vi "SLM_CalibratorOnly1.vi"() -> ()   [LabVIEW 2011]
uses:
  <vilib>/userDefined/High Color/IMAQdx.ctl
  <vilib>/vision/driver/NI_Vision_Acquisition_Software.lvlib
  <vilib>/vision/NI_Vision_Development_Module.lvlib
panel:
  in  "Step:":i32=4
  in  "Boolean":bool caption="SLM1"
  in  "path":path=path "C:/Users/Lab541/Documents/BAUL - TRASH/070214_SLM2" caption="Folder to save data"
  in  "STOP":bool
  out "CCD":T1(plugin-control)
  out "SupportFiles path":path
  in  "Ready?\nCalibrate!":bool caption="Stop (F)"
  in  "Active2":bool=TRUE caption="Hide/Show (Show)"
  in  "Active1":bool=TRUE caption="Hide/Show (Show)"
  in  "Yc1":dbl(slide)=1.3147410358565736 scale=0.0..10.0
  in  "Yf1:":dbl(slide)=2.8685258964143427 caption="Fine:" scale=0.0..10.0
  in  "Xc1":dbl(slide)=9.664429530201343 caption="X position" scale=0.0..10.0
  in  "Xf1:":dbl(slide)=9.664429530201343 caption="Fine:" scale=0.0..10.0
  out "Yi1":dbl caption="Y position"
  out "Xi1":dbl
  in  "Xc2":dbl(slide)=1.4429530201342282 caption="X position" scale=0.0..10.0
  in  "Xf2:":dbl(slide)=6.10738255033557 caption="Fine:" scale=0.0..10.0
  out "Xi2":dbl
  in  "Yf2:":dbl(slide)=5.467625899280575 caption="Fine:" scale=0.0..10.0
  in  "Yc2":dbl(slide)=3.598326359832636 scale=0.0..10.0
  out "Yi2":dbl caption="Y position"
  out "CGH_x\nSLM1":T1(plugin-control)
  out "CGH_y\nSLM2":T1(plugin-control)
  in  "Gradient1":bool
  in  "Gradient2":bool
  out "Status:":string
  in  "Label:":string
  out "Images done":dbl(slide) scale=0.0..256.0
  # "SLM2"
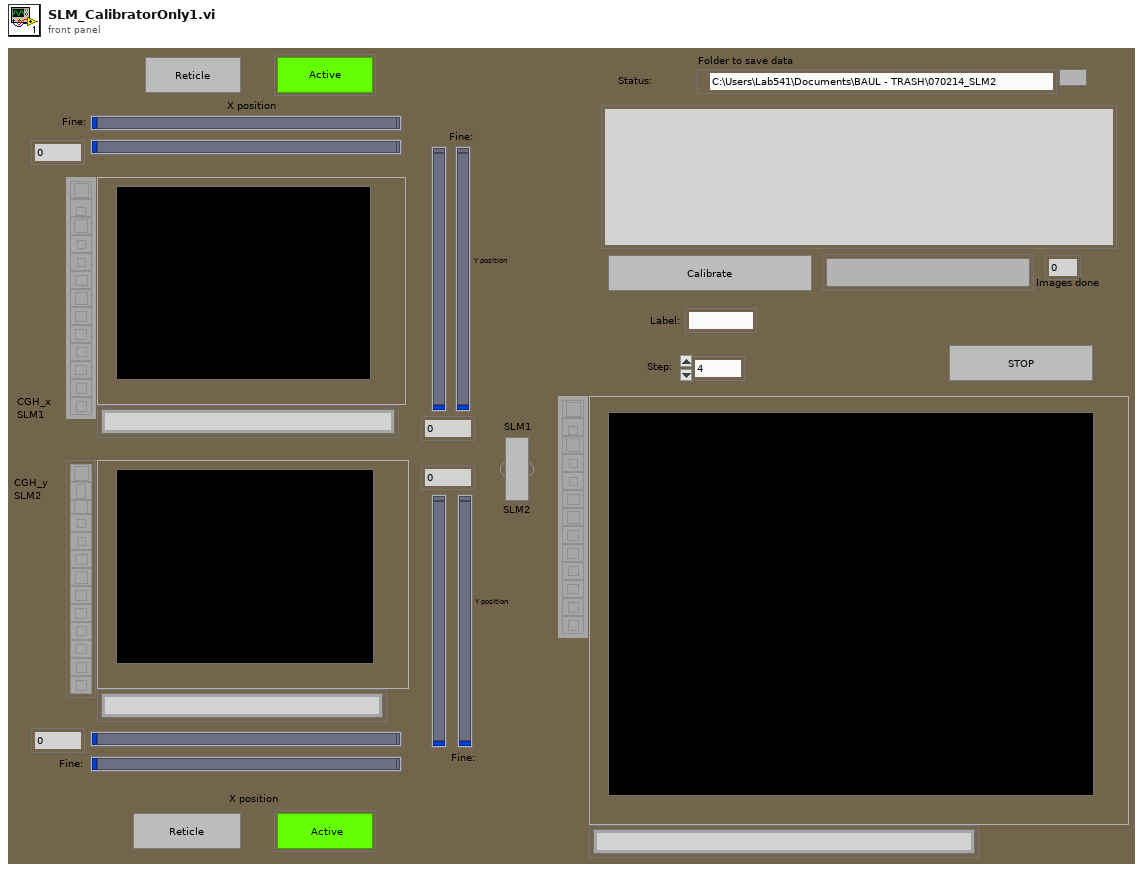
[diagram p1: front panel]
types:
  T1 = typedef "IMAQ Image.ctl" = refnum<image>
  T2 = typedef "IMAQdx.ctl" = refnum<k21>
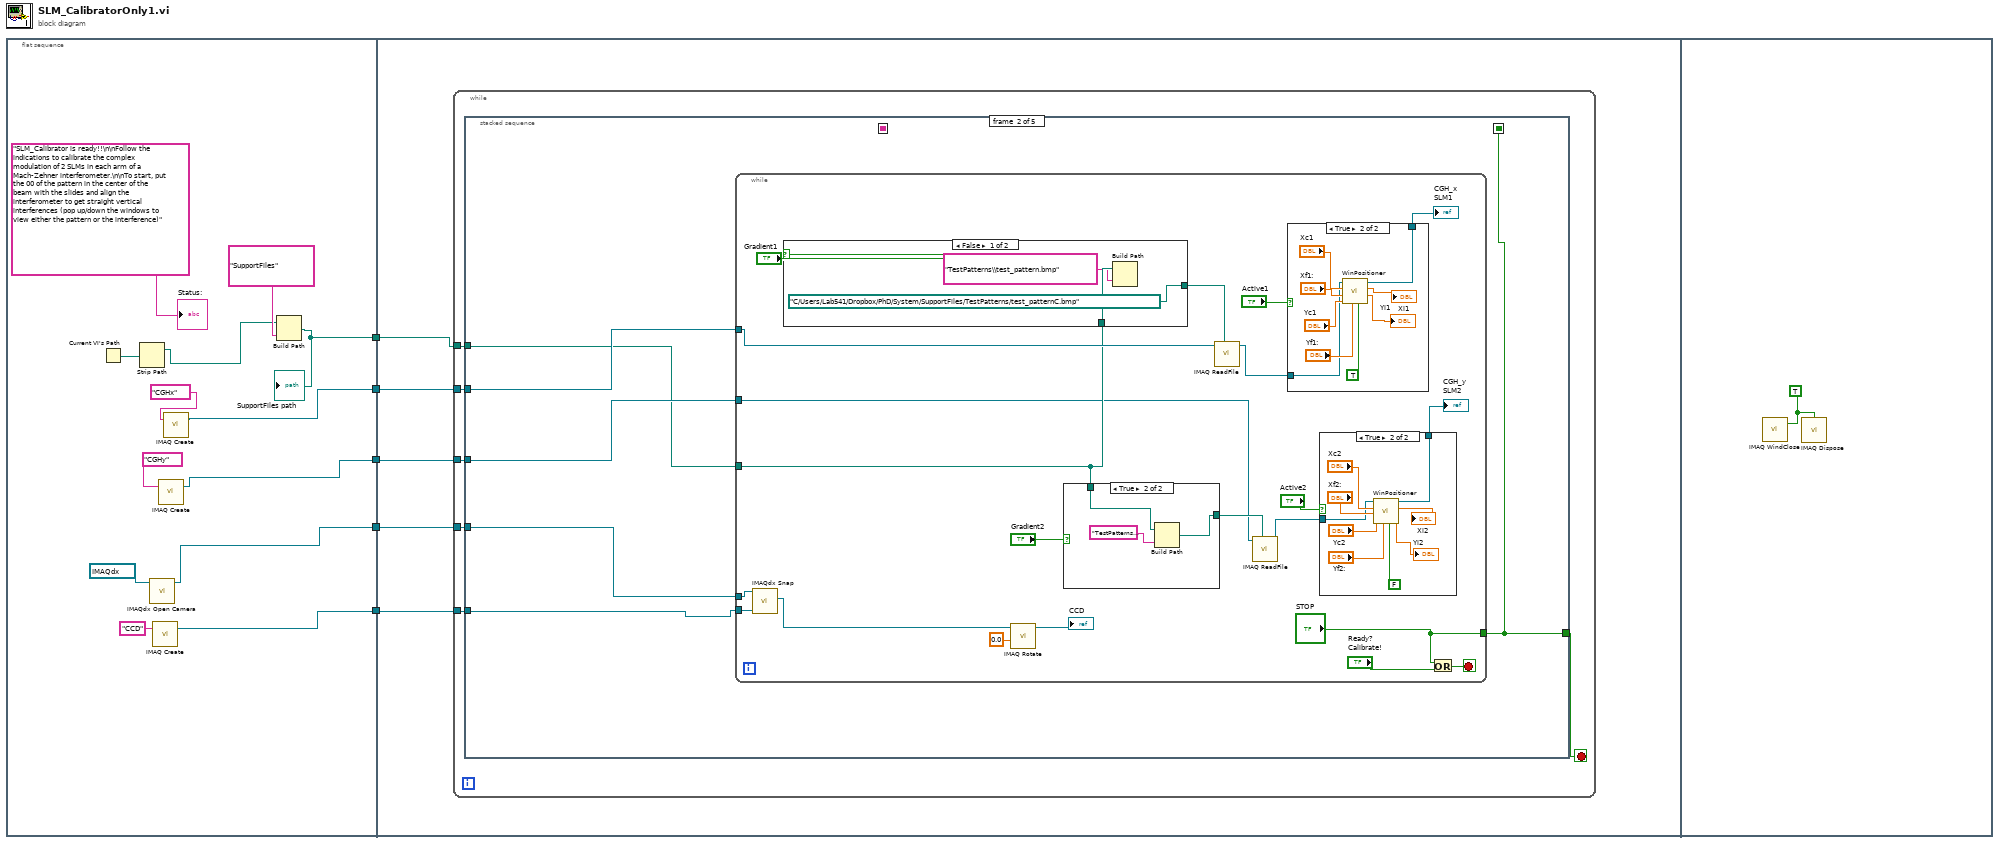
[diagram p0: block diagram]
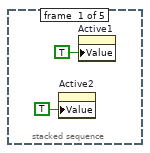
[diagram p2: hidden frame]
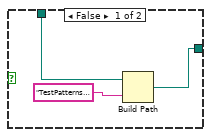
[diagram p3: hidden frame]
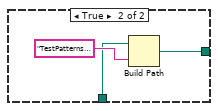
[diagram p4: hidden frame]
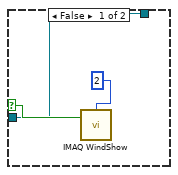
[diagram p5: hidden frame]
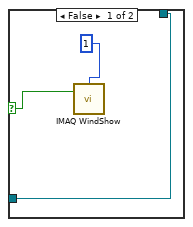
[diagram p6: hidden frame]
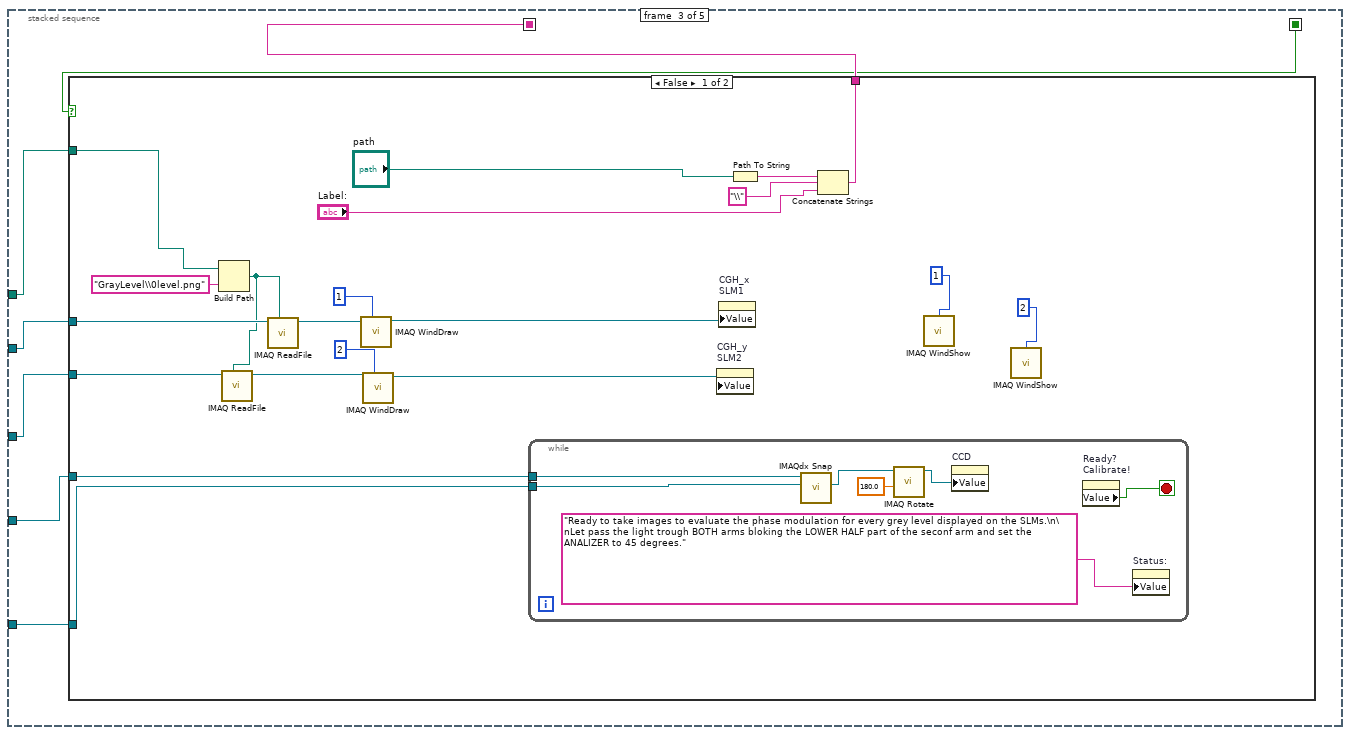
[diagram p7: hidden frame]
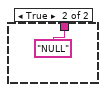
[diagram p8: hidden frame]
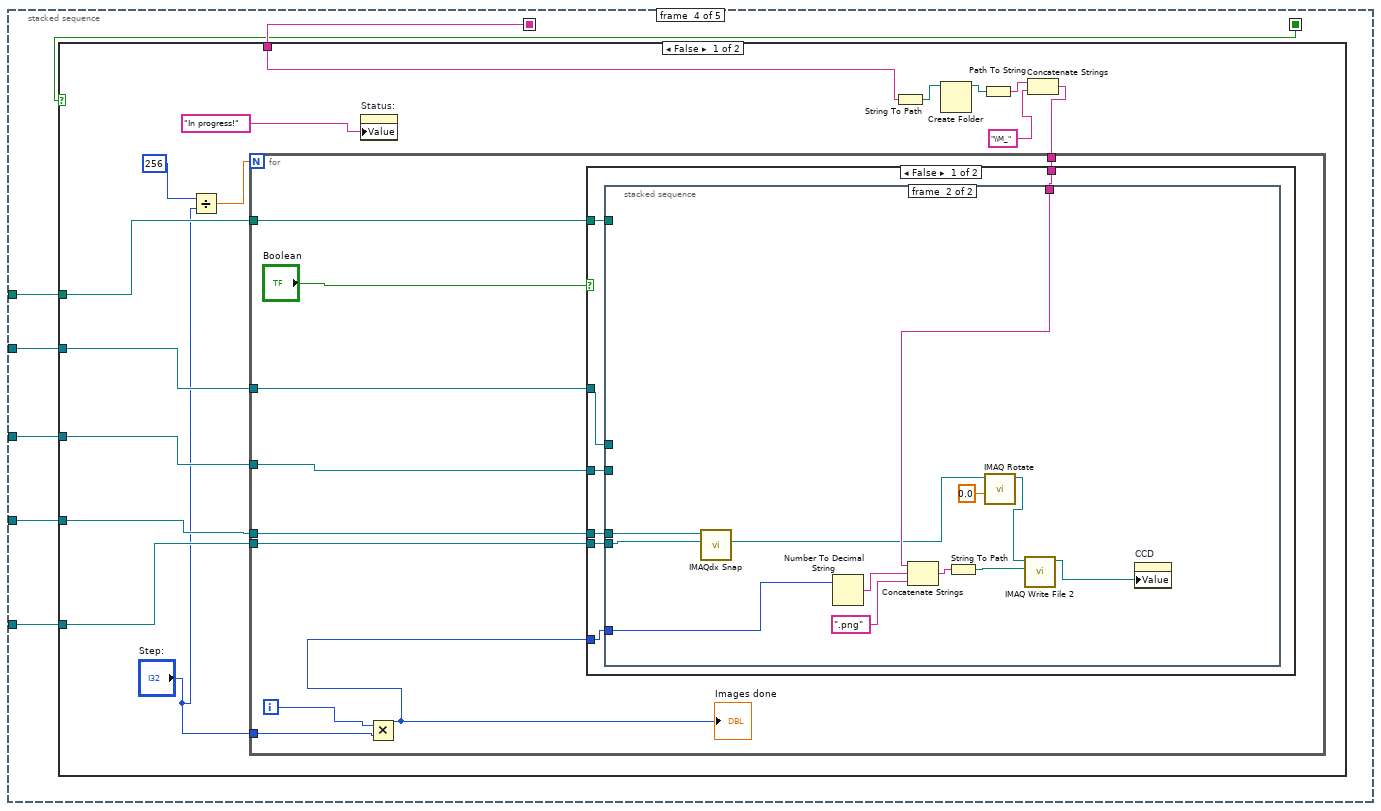
[diagram p9: hidden frame]
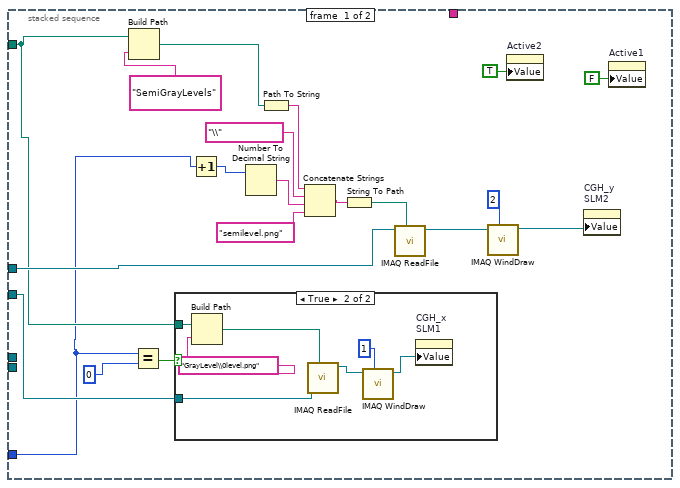
[diagram p10: hidden frame]
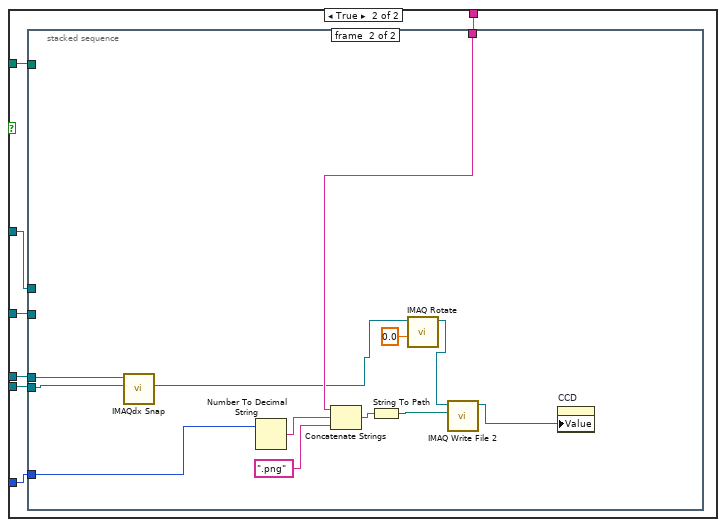
[diagram p12: hidden frame]
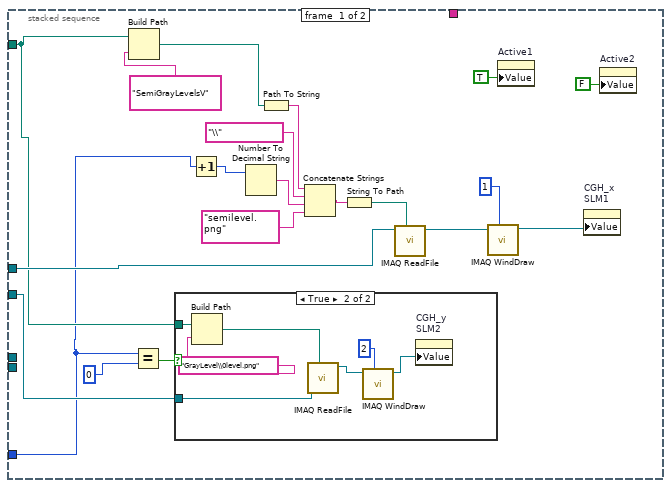
[diagram p13: hidden frame]
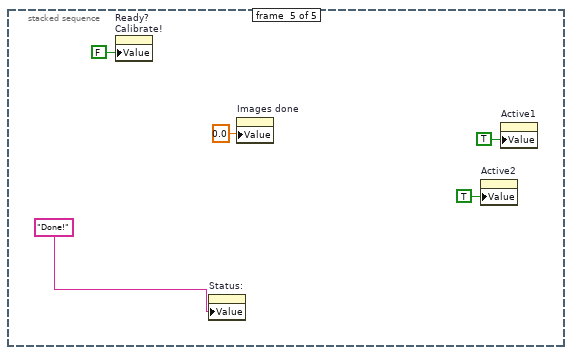
[diagram p16: hidden frame]
diagram:
  n1 = flat-sequence {
    tunnel: [w10] -> w5
    tunnel: [w9] -> w4
    tunnel: [w8] -> w3
    tunnel: [w7] -> w2
    tunnel: [w6] -> w1
    tunnel: w5 -> [w23]
    tunnel: w4 -> [w22]
    tunnel: w3 -> [w21]
    tunnel: w2 -> [w20]
    tunnel: w1 -> [w19]
    frame #0 {
      n2 = Current VI's Path() -> (path=w14:path)
      n3 = Strip Path(path=w14) -> (stripped path=w15:path)  [unwired: 1 out]
      n4 = call <vilib>:"IMAQdx Open Camera.vi"("Session In"=T2 "cam0") -> ("Session Out"=w7:T2)  [unwired: 9 in, 1 out]
      n5 = call "IMAQ Create"("Image Name"="CCD") -> ("New Image"=w6:T1)  [unwired: 4 in, 1 out]
      n6 = call "IMAQ Create"("Image Name"="CGHy") -> ("New Image"=w8:T1)  [unwired: 4 in, 1 out]
      n7 = call "IMAQ Create"("Image Name"="CGHx") -> ("New Image"=w9:T1)  [unwired: 4 in, 1 out]
      n8 = Build Path(base path=w15, name or relative path="SupportFiles") -> (appended path=w10:path)
      "SupportFiles path" <- w10
      "Status:" <- "SLM_Calibrator is ready!!\n\nFollow the indications to calibrate the complex modulation of 2 SLMs in each arm of a Mach-Zehner interferometer.\n\nTo start, put the 00 of the pattern in the center of the beam with the slides and align the interferometer to get straight vertical interferences (pop up/down the windows to view either the pattern or the interference)" ("String")
    }
    frame #1 {
      n9 = while {
        tunnel: w22 -> [w29]
        tunnel: w21 -> [w28]
        tunnel: w19 -> [w27]
        tunnel: w20 -> [w26]
        tunnel: w23 -> [w25]
        stop <- w24 stop-if-true
        n10 = stacked-sequence {
          seq-local: [_ _ w101 _ _] -> [_ _ _ w134 _]
          seq-local: [_ w32 _ _ _] -> [_ _ w95 w130 _]
          tunnel: w28 -> [_ w36 w97 w135 _]
          tunnel: w29 -> [_ w37 w98 w136 _]
          tunnel: w25 -> [_ w35 w99 w133 _]
          tunnel: w27 -> [_ w34 w100 w131 _]
          tunnel: w26 -> [_ w33 w96 w132 _]
          tunnel: [_ w32 _ _ _] -> w24
          frame #0 {
            n11 = property on="Active2" class="Bool (strict)"("Value"=TRUE ("Active1")) -> ()  [unwired: 2 in, 2 out]
            n12 = property on="Active1" class="Bool (strict)"("Value"=TRUE ("Active1")) -> ()  [unwired: 2 in, 2 out]
          }
          frame #1 {
            n13 = while {
              tunnel: w33 -> [w58]
              tunnel: w34 -> [w57]
              tunnel: w37 -> [w51]
              tunnel: w36 -> [w42]
              tunnel: w35 -> [w46]
              tunnel: ["STOP"] -> w32
              stop <- w55 stop-if-true
              n14 = call <vilib>:"IMAQdx Snap.vi"("Image In"=w57, "Session In"=w58) -> ("Image Out"=w40:T1)  [unwired: 7 in, 2 out]
              n15 = case shown="False" "Gradient1" {
                tunnel: w46 -> [w67 w69]
                tunnel: [path "C:/Users/Lab541/Dropbox/PhD/System/SupportFiles/TestPatterns/test_patternC.bmp" ("appended path") w68] -> w47
                frame False {
                  n16 = Build Path(base path=w67, name or relative path="TestPatterns\\test_pattern.bmp") -> ()  [unwired: 1 out]
                }
                frame True {
                  n17 = Build Path(base path=w69, name or relative path="TestPatterns\\test_pattern2V.png") -> (appended path=w68:path)
                }
              }
              n18 = call "IMAQ Rotate"("Angle (degrees)"=sgl 0.0, "Image Src"=w40) -> ("Image Dst Out"=→"CCD":T1)  [unwired: 8 in, 1 out]
              n19 = case shown="True" "Gradient2" {
                tunnel: [w60 w62] -> w44
                tunnel: w46 -> [w59 w63]
                frame False {
                  n20 = Build Path(base path=w59, name or relative path="TestPatterns\\test_pattern.bmp") -> (appended path=w60:path)
                }
                frame True {
                  n21 = Build Path(base path=w63, name or relative path="TestPatterns\\test_pattern2.png") -> (appended path=w62:path)
                }
              }
              n22 = call "IMAQ ReadFile"("File Path"=w47, "Image"=w51) -> ("Image Out"=w43:T1)  [unwired: 5 in, 4 out]
              n23 = call "IMAQ ReadFile"("File Path"=w44, "Image"=w42) -> ("Image Out"=w52:T1)  [unwired: 5 in, 4 out]
              n24 = case shown="True" "Active1" {
                selector: "Active1" -> [w85 _]
                tunnel: [w83 w86] -> w50
                tunnel: w43 -> [w83 w87]
                frame False {
                  n25 = call "IMAQ WindShow"("Hide/Show (Show)"=w85, "Window Number (0...15)"=1) -> ()  [unwired: 4 in, 3 out]
                }
                frame True {
                  n26 = call "WinPositioner.vi"("Image"=w87, "X position"="Xc1", "Fine X position"="Xf1:", "Y position"="Yc1", "Fine Y position"="Yf1:", "Display?"=TRUE) -> ("CGH_x"=w86:T1, "X position"=→"Xi1":dbl, "Y position"=→"Yi1":dbl)  [unwired: 2 in]
                }
              }
              "CGH_x\nSLM1" <- w50
              n27 = case shown="True" "Active2" {
                selector: "Active2" -> [w73 _]
                tunnel: [w71 w74] -> w53
                tunnel: w52 -> [w71 w75]
                frame False {
                  n28 = call "IMAQ WindShow"("Hide/Show (Show)"=w73, "Window Number (0...15)"=2) -> ()  [unwired: 4 in, 3 out]
                }
                frame True {
                  n29 = call "WinPositioner.vi"("Image"=w75, "X position"="Xc2", "Fine X position"="Xf2:", "Y position"="Yc2", "Fine Y position"="Yf2:", "Display?"=FALSE) -> ("CGH_x"=w74:T1, "X position"=→"Xi2":dbl, "Y position"=→"Yi2":dbl)  [unwired: 2 in]
                }
              }
              "CGH_y\nSLM2" <- w53
              n30 = Or(x="STOP", y="Ready?\nCalibrate!") -> (x .or. y?=w55:bool)
            }
          }
          frame #2 {
            n31 = case shown="False" w95 {
              tunnel: [w118 "NULL"] -> w101
              tunnel: w100 -> [w117 _]
              tunnel: w99 -> [w112 _]
              tunnel: w98 -> [w107 _]
              tunnel: w97 -> [w104 _]
              tunnel: w96 -> [w103 _]
              frame False {
                n32 = Build Path(base path=w112, name or relative path="GrayLevel\\0level.png") -> (appended path=w105:path)
                n33 = call "IMAQ ReadFile"("File Path"=w105, "Image"=w104) -> ("Image Out"=w106:T1)  [unwired: 5 in, 4 out]
                n34 = call "IMAQ ReadFile"("File Path"=w105, "Image"=w107) -> ("Image Out"=w108:T1)  [unwired: 5 in, 4 out]
                n35 = call "IMAQ WindDraw"("Window Number (0...15)"=1, "Image"=w108) -> ("Image Out (duplicate)"=w113:T1)  [unwired: 8 in, 1 out]
                n36 = call "IMAQ WindDraw"("Window Number (0...15)"=2, "Image"=w106) -> ("Image Out (duplicate)"=w109:T1)  [unwired: 8 in, 1 out]
                n37 = while {
                  tunnel: w103 -> [w127]
                  tunnel: w117 -> [w126]
                  stop <- w125 stop-if-true
                  n38 = call <vilib>:"IMAQdx Snap.vi"("Image In"=w126, "Session In"=w127) -> ("Image Out"=w123:T1)  [unwired: 7 in, 2 out]
                  n39 = call "IMAQ Rotate"("Angle (degrees)"=sgl 180.0, "Image Src"=w123) -> ("Image Dst Out"=w122:T1)  [unwired: 8 in, 1 out]
                  n40 = property on="CCD" class="ImageControl"("Value"=w122) -> ()  [unwired: 2 in, 2 out]
                  n41 = property on="Ready?\nCalibrate!" class="Bool (strict)"() -> ("Value"=w125:bool)  [unwired: 2 in, 2 out]
                  n42 = property on="Status:" class="Str"("Value"="Ready to take images to evaluate the phase modulation for every grey level displayed on the SLMs.\n\nLet pass the light trough BOTH arms bloking the LOWER HALF part of the seconf arm and set the ANALIZER to 45 degrees." ("message")) -> ()  [unwired: 2 in, 2 out]
                }
                n43 = property on="CGH_y\nSLM2" class="ImageControl"("Value"=w109) -> ()  [unwired: 2 in, 2 out]
                n44 = property on="CGH_x\nSLM1" class="ImageControl"("Value"=w113) -> ()  [unwired: 2 in, 2 out]
                n45 = Path To String(path="path") -> (string=w121:string)
                n46 = Concatenate Strings(w121, "\\" ("string"), "Label:") -> (w118:string)
                n47 = call "IMAQ WindShow"("Window Number (0...15)"=1) -> ()  [unwired: 5 in, 3 out]
                n48 = call "IMAQ WindShow"("Window Number (0...15)"=2) -> ()  [unwired: 5 in, 3 out]
              }
              frame True {
              }
            }
          }
          frame #3 {
            n49 = case shown="False" w130 {
              tunnel: w136 -> [w151 _]
              tunnel: w135 -> [w150 _]
              tunnel: w134 -> [w144 _]
              tunnel: w133 -> [w142 _]
              tunnel: w132 -> [w141 _]
              tunnel: w131 -> [w143 _]
              frame False {
                n50 = Divide(x=256, y="Step:") -> (x/y=w138:dbl)
                n51 = property on="Status:" class="Str"("Value"="In progress!" ("Status")) -> ()  [unwired: 2 in, 2 out]
                n52 = String To Path(string=w144) -> (path=w148:path)
                n53 = Create Folder(path (use dialog)=w148) -> (created path=w147:path)  [unwired: 2 in, 2 out]
                n54 = Path To String(path=w147) -> (string=w146:string)
                n55 = Concatenate Strings(w146, "\\M_") -> (w137:string)
                n56 = for {
                  N: w138 -> [_]
                  tunnel: w151 -> [w161]
                  tunnel: w150 -> [w160]
                  tunnel: w137 -> [w159]
                  tunnel: w142 -> [w158]
                  tunnel: w141 -> [w157]
                  tunnel: w143 -> [w156]
                  tunnel: "Step:" -> [w152]
                  i -> [w155]
                  n57 = Multiply(x=w155, y=w152) -> (x*y=w154:i32)
                  "Images done" <- w154
                  n58 = case shown="False" "Boolean" {
                    tunnel: w161 -> [w162 w213]
                    tunnel: w160 -> [w168 w212]
                    tunnel: w159 -> [w167 w209]
                    tunnel: w158 -> [w166 w214]
                    tunnel: w157 -> [w165 w211]
                    tunnel: w156 -> [w164 w210]
                    tunnel: w154 -> [w163 w208]
                    frame False {
                      n59 = stacked-sequence {
                        tunnel: w163 -> [w171 w203]
                        tunnel: w162 -> [w188 _]
                        tunnel: w168 -> [w173 _]
                        tunnel: w167 -> [_ w202]
                        tunnel: w166 -> [w174 _]
                        tunnel: w165 -> [_ w201]
                        tunnel: w164 -> [_ w200]
                        frame #0 {
                          n60 = Build Path(base path=w174, name or relative path="SemiGrayLevels") -> (appended path=w175:path)
                          n61 = Equal?(x=w171, y=0) -> (x = y?=w178:bool)
                          n62 = case shown="True" w178 {
                            tunnel: w173 -> [_ w193]
                            tunnel: w174 -> [_ w192]
                            frame False {
                            }
                            frame True {
                              n63 = Build Path(base path=w192, name or relative path="GrayLevel\\0level.png") -> (appended path=w190:path)
                              n64 = call "IMAQ ReadFile"("File Path"=w190, "Image"=w193) -> ("Image Out"=w195:T1)  [unwired: 5 in, 4 out]
                              n65 = call "IMAQ WindDraw"("Window Number (0...15)"=1, "Image"=w195) -> ("Image Out (duplicate)"=w189:T1)  [unwired: 8 in, 1 out]
                              n66 = property on="CGH_x\nSLM1" class="ImageControl"("Value"=w189) -> ()  [unwired: 2 in, 2 out]
                            }
                          }
                          n67 = Increment(x=w171) -> (x+1=w182:i32)
                          n68 = Number To Decimal String(number=w182) -> (decimal integer string=w183:string)  [unwired: 1 in]
                          n69 = Path To String(path=w175) -> (string=w184:string)
                          n70 = Concatenate Strings(w184, "\\", w183, "semilevel.png") -> (w180:string)
                          n71 = String To Path(string=w180) -> (path=w179:path)
                          n72 = call "IMAQ ReadFile"("File Path"=w179, "Image"=w188) -> ("Image Out"=w187:T1)  [unwired: 5 in, 4 out]
                          n73 = call "IMAQ WindDraw"("Window Number (0...15)"=2, "Image"=w187) -> ("Image Out (duplicate)"=w172:T1)  [unwired: 8 in, 1 out]
                          n74 = property on="Active2" class="Bool (strict)"("Value"=TRUE ("Active1")) -> ()  [unwired: 2 in, 2 out]
                          n75 = property on="CGH_y\nSLM2" class="ImageControl"("Value"=w172) -> ()  [unwired: 2 in, 2 out]
                          n76 = property on="Active1" class="Bool (strict)"("Value"=FALSE ("Active2")) -> ()  [unwired: 2 in, 2 out]
                        }
                        frame #1 {
                          n77 = call <vilib>:"IMAQdx Snap.vi"("Image In"=w200, "Session In"=w201) -> ("Image Out"=w197:T1)  [unwired: 7 in, 2 out]
                          n78 = Number To Decimal String(number=w203) -> (decimal integer string=w205:string)  [unwired: 1 in]
                          n79 = Concatenate Strings(w202, w205, ".png") -> (w207:string)
                          n80 = String To Path(string=w207) -> (path=w204:path)
                          n81 = call "IMAQ Rotate"("Angle (degrees)"=sgl 0.0, "Image Src"=w197) -> ("Image Dst Out"=w196:T1)  [unwired: 8 in, 1 out]
                          n82 = call-poly "IMAQ Write File 2"("File Path"=w204, "Image"=w196) -> ("Image Out (duplicate)"=w199:T1)  [unwired: 8 in, 1 out]
                          n83 = property on="CCD" class="ImageControl"("Value"=w199) -> ()  [unwired: 2 in, 2 out]
                        }
                      }
                    }
                    frame True {
                      n84 = stacked-sequence {
                        tunnel: w208 -> [w217 w249]
                        tunnel: w213 -> [w234 _]
                        tunnel: w212 -> [w219 _]
                        tunnel: w209 -> [_ w248]
                        tunnel: w214 -> [w220 _]
                        tunnel: w211 -> [_ w247]
                        tunnel: w210 -> [_ w246]
                        frame #0 {
                          n85 = Build Path(base path=w220, name or relative path="SemiGrayLevelsV") -> (appended path=w221:path)
                          n86 = Equal?(x=w217, y=0) -> (x = y?=w224:bool)
                          n87 = case shown="True" w224 {
                            tunnel: w219 -> [_ w239]
                            tunnel: w220 -> [_ w238]
                            frame False {
                            }
                            frame True {
                              n88 = Build Path(base path=w238, name or relative path="GrayLevel\\0level.png") -> (appended path=w236:path)
                              n89 = call "IMAQ ReadFile"("File Path"=w236, "Image"=w239) -> ("Image Out"=w241:T1)  [unwired: 5 in, 4 out]
                              n90 = call "IMAQ WindDraw"("Window Number (0...15)"=2, "Image"=w241) -> ("Image Out (duplicate)"=w235:T1)  [unwired: 8 in, 1 out]
                              n91 = property on="CGH_y\nSLM2" class="ImageControl"("Value"=w235) -> ()  [unwired: 2 in, 2 out]
                            }
                          }
                          n92 = Increment(x=w217) -> (x+1=w228:i32)
                          n93 = Number To Decimal String(number=w228) -> (decimal integer string=w229:string)  [unwired: 1 in]
                          n94 = Path To String(path=w221) -> (string=w230:string)
                          n95 = Concatenate Strings(w230, "\\", w229, "semilevel.png") -> (w226:string)
                          n96 = String To Path(string=w226) -> (path=w225:path)
                          n97 = call "IMAQ ReadFile"("File Path"=w225, "Image"=w234) -> ("Image Out"=w233:T1)  [unwired: 5 in, 4 out]
                          n98 = call "IMAQ WindDraw"("Window Number (0...15)"=1, "Image"=w233) -> ("Image Out (duplicate)"=w218:T1)  [unwired: 8 in, 1 out]
                          n99 = property on="Active1" class="Bool (strict)"("Value"=TRUE ("Active1")) -> ()  [unwired: 2 in, 2 out]
                          n100 = property on="CGH_x\nSLM1" class="ImageControl"("Value"=w218) -> ()  [unwired: 2 in, 2 out]
                          n101 = property on="Active2" class="Bool (strict)"("Value"=FALSE ("Active2")) -> ()  [unwired: 2 in, 2 out]
                        }
                        frame #1 {
                          n102 = call <vilib>:"IMAQdx Snap.vi"("Image In"=w246, "Session In"=w247) -> ("Image Out"=w243:T1)  [unwired: 7 in, 2 out]
                          n103 = Number To Decimal String(number=w249) -> (decimal integer string=w251:string)  [unwired: 1 in]
                          n104 = Concatenate Strings(w248, w251, ".png") -> (w253:string)
                          n105 = String To Path(string=w253) -> (path=w250:path)
                          n106 = call "IMAQ Rotate"("Angle (degrees)"=sgl 0.0, "Image Src"=w243) -> ("Image Dst Out"=w242:T1)  [unwired: 8 in, 1 out]
                          n107 = call-poly "IMAQ Write File 2"("File Path"=w250, "Image"=w242) -> ("Image Out (duplicate)"=w245:T1)  [unwired: 8 in, 1 out]
                          n108 = property on="CCD" class="ImageControl"("Value"=w245) -> ()  [unwired: 2 in, 2 out]
                        }
                      }
                    }
                  }
                }
              }
              frame True {
              }
            }
          }
          frame #4 {
            n109 = property on="Ready?\nCalibrate!" class="Bool (strict)"("Value"=FALSE ("Ready?\nCalibrate!")) -> ()  [unwired: 2 in, 2 out]
            n110 = property on="Status:" class="Str"("Value"="Done!") -> ()  [unwired: 2 in, 2 out]
            n111 = property on="Images done" class="Slide (strict)"("Value"=0.0 ("Images done")) -> ()  [unwired: 2 in, 2 out]
            n112 = property on="Active2" class="Bool (strict)"("Value"=TRUE ("Active1")) -> ()  [unwired: 2 in, 2 out]
            n113 = property on="Active1" class="Bool (strict)"("Value"=TRUE ("Active1")) -> ()  [unwired: 2 in, 2 out]
          }
        }
      }
    }
    frame #2 {
      w259 = TRUE ("Close All Windows (False)")
      n114 = call "IMAQ WindClose"("Close All Windows (False)"=w259) -> ()  [unwired: 5 in, 1 out]
      n115 = call "IMAQ Dispose"("All Images? (No)"=w259) -> ()  [unwired: 5 in, 1 out]
    }
  }
